vi "Autonomous Logging 2017.vi"   [LabVIEW 2016]
uses:
  Global Variables/Autonomous Exec Info.vi
  Global Variables/Sensor Data.vi
  Subsystems/Drive and Climb SS/Drive and Climb Logging Values.vi
types:
  T1 = typedef "Autonomous Command Names.ctl" = enum16{"No Op", "Command Drive+Climb Shift", "Command Wait", "Command Deliver Gear", "Command Buffer", "Command Drive Path", "Command Drive Time", "Command Shoot", "Command Turn to Heading", "Command Run Conveyor", "Command Spinup Shooter", "Command Deliver Gear Front", "Command Toggle Intake Rotation", "DO NOT USE", "Command Agitate Hopper", "Command Pre-Buffer", "Command Turn to Target", "Command Deliver Gear with Safety", "Command Drive Time with IMU", "Command Drive to Encoders"}
  T2 = cluster{"Param 1":dbl, "Param 2":dbl, "Autonomous Command Name":T1, "Concurrent":bool, "Param 3":dbl, "Param 4":string}
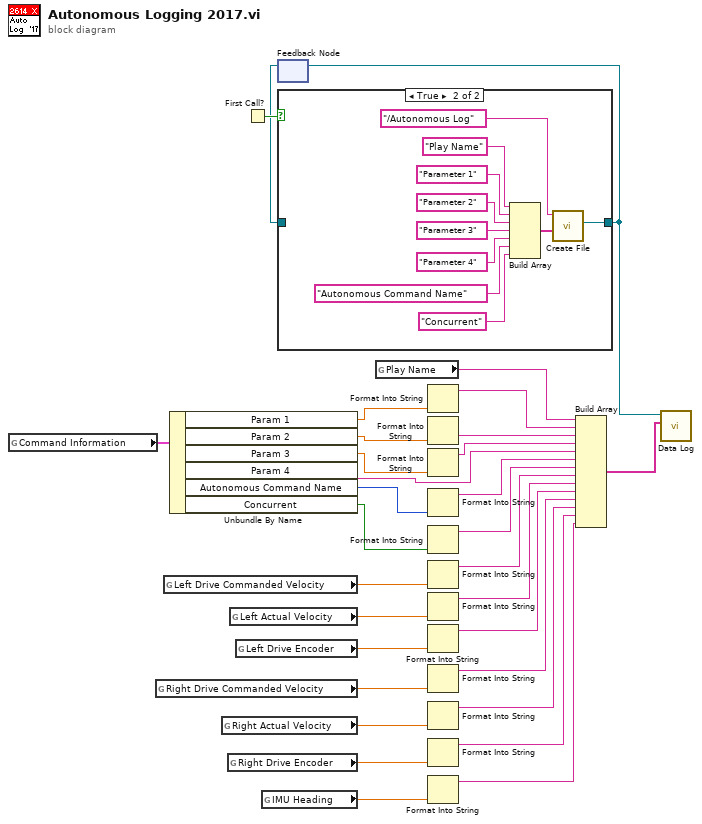
[diagram p0: block diagram]
diagram:
  n1 = global read "Autonomous Exec Info.vi" "Command Information"() -> (w28:T2)
  n2 = global read "Drive and Climb Logging Values.vi" "Right Drive Commanded Velocity"() -> (w4:dbl)
  n3 = global read "Drive and Climb Logging Values.vi" "Left Drive Commanded Velocity"() -> (w7:dbl)
  n4 = Unbundle By Name(w28) -> ("Param 1"=w27:dbl, "Param 2"=w25:dbl, "Param 3"=w22:dbl, "Param 4"=w20:string, "Autonomous Command Name"=w24:T1, "Concurrent"=w19:bool)
  n5 = global read "Drive and Climb Logging Values.vi" "Right Actual Velocity"() -> (w3:dbl)
  n6 = global read "Sensor Data.vi" "Right Drive Encoder"() -> (w2:dbl)
  n7 = global read "Drive and Climb Logging Values.vi" "Left Actual Velocity"() -> (w6:dbl)
  n8 = global read "Sensor Data.vi" "Left Drive Encoder"() -> (w5:dbl)
  n9 = First Call?() -> (First Call?: T/F=w31:bool)
  n10 = global read "Sensor Data.vi" "IMU Heading"() -> (w1:dbl)
  n11 = feedback #1() -> (w30:refnum<file>)  [unwired: 1 in]
  n12 = case shown="True" w31 {
    tunnel: [w32 w33] -> w29
    tunnel: w30 -> [w32 _]
    frame False {
    }
    frame True {
      n13 = Build Array("Play Name" ("string"), "Parameter 1" ("string"), "Parameter 2" ("string"), "Parameter 3" ("string"), "Parameter 4" ("string"), "Autonomous Command Name" ("string"), "Concurrent" ("string")) -> (w42:string[])
      n14 = call "Create File.vi"("Column Titles"=w42, "File Name"="/Autonomous Log" ("string")) -> ("File Reference Out"=w33:refnum<file>)  [unwired: 9 in]
    }
  }
  n15 = feedback-in #1(w29) -> ()
  n16 = global read "Autonomous Exec Info.vi" "Play Name"() -> (w15:string)
  n17 = Format Into String(w27) -> (resulting string=w26:string)  [unwired: 3 in, 1 out]
  n18 = Format Into String(w25) -> (resulting string=w23:string)  [unwired: 3 in, 1 out]
  n19 = Format Into String(w22) -> (resulting string=w21:string)  [unwired: 3 in, 1 out]
  n20 = Format Into String(w24) -> (resulting string=w17:string)  [unwired: 3 in, 1 out]
  n21 = Format Into String(w19) -> (resulting string=w18:string)  [unwired: 3 in, 1 out]
  n22 = Format Into String(w7) -> (resulting string=w14:string)  [unwired: 3 in, 1 out]
  n23 = Format Into String(w6) -> (resulting string=w13:string)  [unwired: 3 in, 1 out]
  n24 = Format Into String(w5) -> (resulting string=w12:string)  [unwired: 3 in, 1 out]
  n25 = Format Into String(w4) -> (resulting string=w11:string)  [unwired: 3 in, 1 out]
  n26 = Format Into String(w3) -> (resulting string=w10:string)  [unwired: 3 in, 1 out]
  n27 = Format Into String(w2) -> (resulting string=w9:string)  [unwired: 3 in, 1 out]
  n28 = Format Into String(w1) -> (resulting string=w8:string)  [unwired: 3 in, 1 out]
  n29 = Build Array(w15, w26, w23, w21, w20, w17, w18, w14, w13, w12, w11, w10, w9, w8) -> (w16:string[])
  n30 = call "Data Log.vi"("Data In"=w16, "File Reference In"=w29) -> ()  [unwired: 9 in, 1 out]
